vi "Phase Analysis FPGA AI_9215.vi"(4 "Offset":dbl, 6 "NumAI Channels":u32, 8 "error in (no error)":errorcluster, 10 "LVFPGA Data in":fxp<+/-,24,5>[](array[numeric]), 11 "cDAQ data in":waveform(dbl)[](array[waveform])) -> (0 "error out":errorcluster, 1 "Phase Histogram":T1(graph), 2 "Phase Plot":dbl[][](graph), 3 "Waveform Plot":waveform(dbl)[](array[waveform]), 5 "Phase Jitter (ns)":dbl, 7 "Peak Phase (ns)":dbl)   [LabVIEW 2018]
uses:
  <vilib>/measure/matone.llb/Extract Single Tone Information N Chan.vi
  <vilib>/measure/NI_MAPro.lvlib
  <vilib>/Analysis/NI_AALPro.lvlib
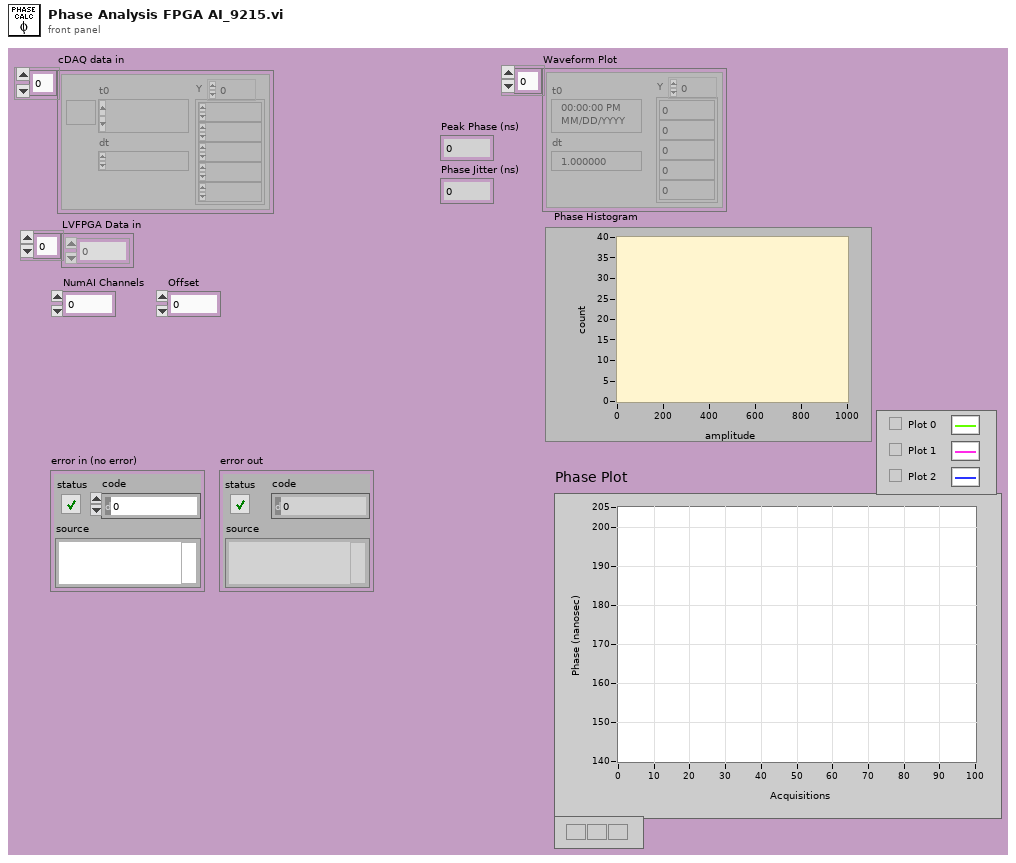
[diagram p1: front panel]
types:
  T1 = cluster{"X Values":dbl[], "Histogram: h(x)":i32[]}
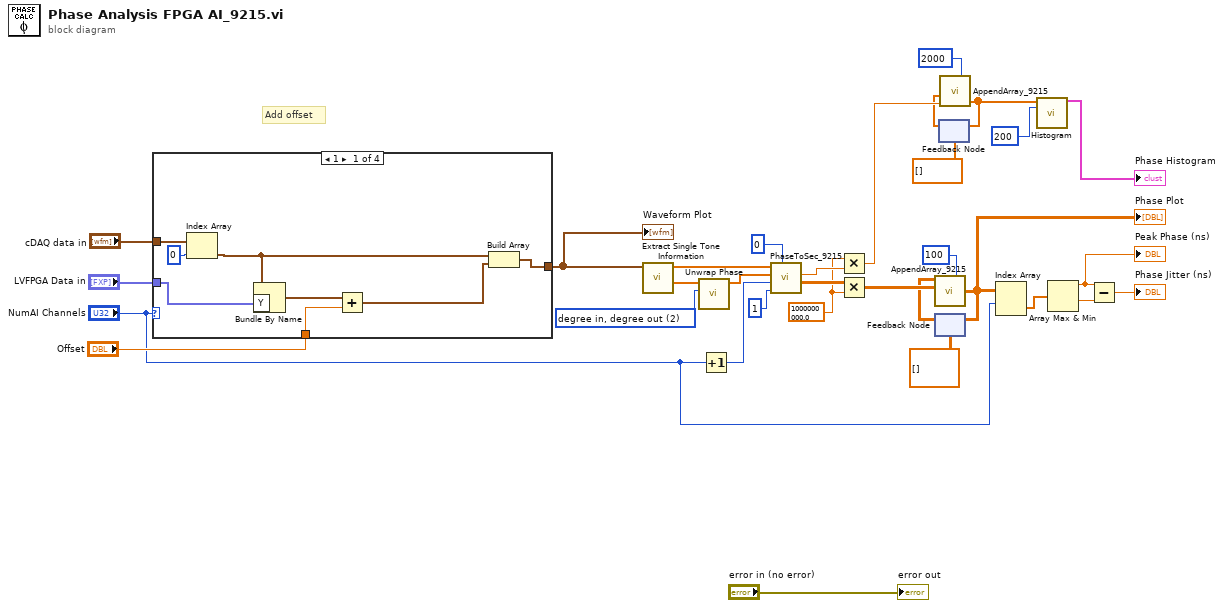
[diagram p0: block diagram]
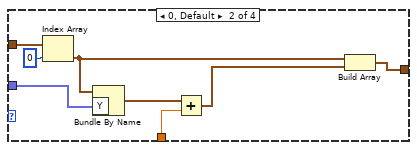
[diagram p2: hidden frame]
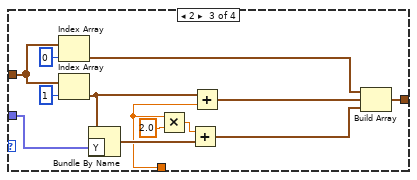
[diagram p3: hidden frame]
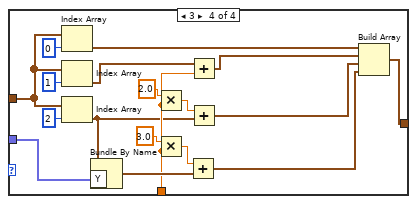
[diagram p4: hidden frame]
diagram:
  w1 = 1000000000.0 ("y")
  w31 = 2 items=["radian in, radian out", "radian in, degree out", "degree in, degree out", "degree in, radian out"] ("phase unit")
  # "Add offset"
  n1 = case shown="1" "NumAI Channels" {
    tunnel: "cDAQ data in" -> [w39 w46 w59 w76]
    tunnel: "Offset" -> [w33 w42 w50 w64]
    tunnel: [w38 w41 w56 w66] -> w5
    tunnel: "LVFPGA Data in" -> [w36 w44 w54 w70]
    frame 1 {
      n2 = Index Array(array=w39, index=0) -> (element=w35:waveform(dbl))
      n3 = Bundle By Name(cluster=w35, "Y"=w36) -> (w37:waveform(dbl))
      n4 = Add(x=w37, y=w33) -> (x+y=w34:waveform(dbl))
      n5 = Build Array(w35, w34) -> (w38:waveform(dbl)[])
    }
    frame 0, Default {
      n6 = Index Array(array=w46, index=0) -> (element=w45:waveform(dbl))
      n7 = Bundle By Name(cluster=w45, "Y"=w44) -> (w43:waveform(dbl))
      n8 = Add(x=w43, y=w42) -> (x+y=w47:waveform(dbl))
      n9 = Build Array(w45, w47) -> (w41:waveform(dbl)[])
    }
    frame 2 {
      n10 = Index Array(array=w59, index=0) -> (element=w58:waveform(dbl))
      n11 = Index Array(array=w59, index=1) -> (element=w55:waveform(dbl))
      n12 = Bundle By Name(cluster=w55, "Y"=w54) -> (w52:waveform(dbl))
      n13 = Multiply(x=w50, y=2.0 ("x")) -> (x*y=w53:dbl)
      n14 = Add(x=w53, y=w52) -> (x+y=w51:waveform(dbl))
      n15 = Add(x=w55, y=w50) -> (x+y=w57:waveform(dbl))
      n16 = Build Array(w58, w57, w51) -> (w56:waveform(dbl)[])
    }
    frame 3 {
      n17 = Index Array(array=w76, index=0) -> (element=w73:waveform(dbl))
      n18 = Index Array(array=w76, index=1) -> (element=w74:waveform(dbl))
      n19 = Index Array(array=w76, index=2) -> (element=w62:waveform(dbl))
      n20 = Bundle By Name(cluster=w62, "Y"=w70) -> (w68:waveform(dbl))
      n21 = Multiply(x=2.0, y=w64) -> (x*y=w63:dbl)
      n22 = Multiply(x=3.0, y=w64) -> (x*y=w67:dbl)
      n23 = Add(x=w67, y=w68) -> (x+y=w65:waveform(dbl))
      n24 = Add(x=w74, y=w64) -> (x+y=w72:waveform(dbl))
      n25 = Add(x=w63, y=w62) -> (x+y=w71:waveform(dbl))
      n26 = Build Array(w73, w72, w71, w65) -> (w66:waveform(dbl)[])
    }
  }
  "Waveform Plot" <- w5
  n27 = call-poly <vilib>:"Extract Single Tone Information.vi"("time signals in"=w5) -> ("detected phases (deg)"=w32:dbl[], "detected frequencies"=w30:dbl[])  [unwired: 5 in, 4 out]
  n28 = call <vilib>:"Unwrap Phase.vi"("phase unit"=w31, "Phase"=w32) -> ("Unwrapped Phase"=w29:dbl[])  [unwired: 8 in, 1 out]
  n29 = Increment(x="NumAI Channels") -> (x+1=w4:u32)
  n30 = call "PhaseToSec_9215.vi"("Reference Channel"=u32 0, "NumAcquisitions"=u32 1, "NumChannels"=w4, "Phases"=w29, "Frequencies"=w30) -> ("Max Phase Difference Array"=w26:dbl[][], "Max Phase Difference"=w27:dbl)  [unwired: 4 in, 1 out]
  n31 = Multiply(x=w1, y=w27) -> (x*y=w19:dbl)
  n32 = Multiply(x=w26, y=w1) -> (x*y=w24:dbl[][])
  n33 = feedback #1(dbl[][] [] ("ArrayOut")) -> (w14:dbl[][])
  n34 = call "AppendArray_9215.vi"("Array Max Size"=100, "2D AppendArr"=w24, "2D ArrayIn"=w14) -> ("2D ArrayOut"=w15:dbl[][])  [unwired: 2 in, 1 out]
  "Phase Plot" <- w15
  n35 = feedback-in #1(w15) -> ()
  n36 = feedback #2(dbl[] []) -> (w11:dbl[])
  n37 = call "AppendArray_9215.vi"("Array Max Size"=2000, "Append Element"=w19, "1D Array In"=w11) -> ("1D Array Out"=w12:dbl[])  [unwired: 2 in, 1 out]
  n38 = feedback-in #2(w12) -> ()
  n39 = Index Array(array=w15, index (row)="NumAI Channels") -> (element=w17:dbl[])  [unwired: 1 in]
  n40 = call "Histogram.vi"("In"=w12, "Intervals"=200) -> ("Histogram"=→"Phase Histogram":T1)  [unwired: 12 in, 1 out]
  n41 = Array Max & Min(array=w17) -> (max value=w21:dbl, min value=w20:dbl)  [unwired: 2 out]
  "Peak Phase (ns)" <- w21
  n42 = Subtract(x=w21, y=w20) -> (x-y=→"Phase Jitter (ns)":dbl)
  "error out" <- "error in (no error)"
